vi "RESTful Qualify Routing Templates.vi"(9 "qualified VI names":string[](array[string]), 10 "relative VI paths":path[](array[path]), 11 "Routing Templates":T1[](array[typedef])) -> (3 "Routing Templates out":T1[](array[typedef]))   [LabVIEW 2020]
uses:
  <vilib>/AppBuilder/AB_Classes/RESTful/AB_RESTful_RoutingTemplate.ctl
  <vilib>/AppBuilder/AB_Classes/RESTful/AB_RESTful_RoutingType.ctl
  <vilib>/AppBuilder/AB_Classes/RESTful/AB_RESTful_HTTPMethodType.ctl
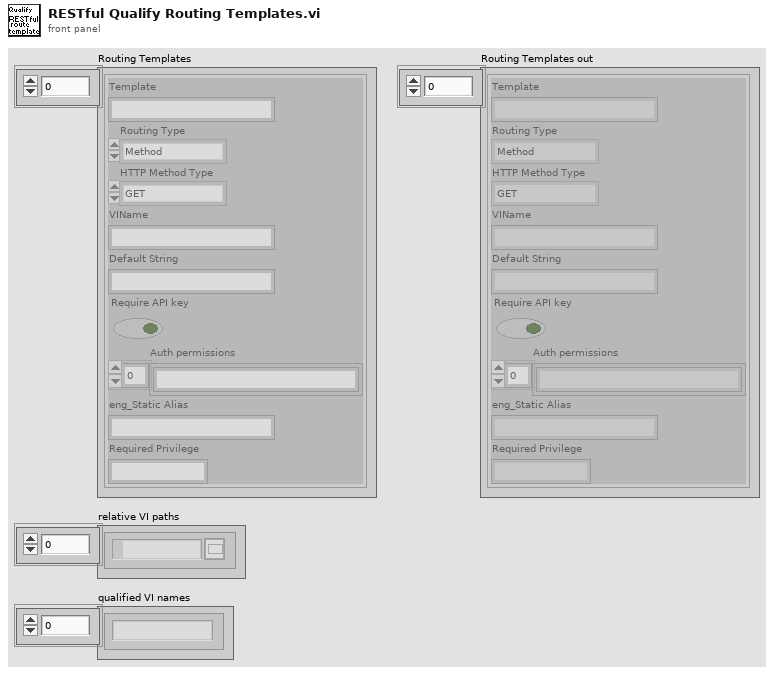
[diagram p1: front panel]
types:
  T1 = typedef "AB_RESTful_RoutingTemplate.ctl" = cluster{"Template":string, "Routing Type":T2, "HTTP Method Type":T3, "VIName":string, "Default String":string, "Require API key":bool, "Auth permissions":string[], "eng_Static Alias":string, "Required Privilege":string}
  T2 = typedef "AB_RESTful_RoutingType.ctl" = enum32{"Method", "Static"}
  T3 = typedef "AB_RESTful_HTTPMethodType.ctl" = enum32{"GET", "POST", "PUT", "DELETE"}
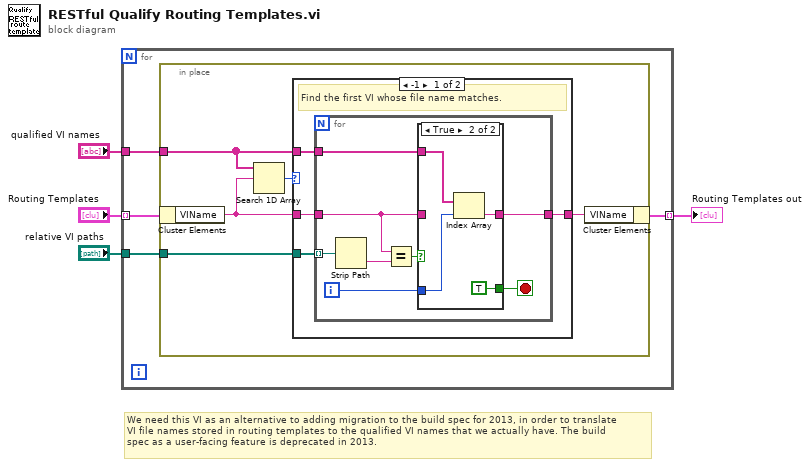
[diagram p0: block diagram]
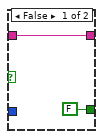
[diagram p2: hidden frame]
diagram:
  # "We need this VI as an alternative to adding migration to the build spec for 2013, in order to translate\nVI file names stored in routing templates to the qualified VI names that we actually have. The build\nspec as a user-facing feature is deprecated in 2013."
  n1 = for {
    tunnel: "Routing Templates" -> [w8] mode=indexing
    tunnel: "qualified VI names" -> [w7]
    tunnel: "relative VI paths" -> [w6]
    tunnel: [w5] -> w4 mode=indexing
    n2 = in-place {
      in-place-border: w7 -> [w9]
      in-place-border: w6 -> [w10]
      n3 = in-place-cluster #1(w8) -> ("VIName"=w12:string)
      n4 = Search 1D Array(1D array=w9, element=w12) -> (index of element=w13:i32)  [unwired: 1 in]
      n5 = case shown="-1" w13 {
        tunnel: w12 -> [w16 w32]
        tunnel: [w14 w32] -> w11
        tunnel: w10 -> [w17 _]
        tunnel: w9 -> [w15 _]
        frame -1 {
          # "Find the first VI whose file name matches."
          n6 = for {
            tunnel: w17 -> [w25] mode=indexing
            tunnel: w16 -> [w19]
            tunnel: w15 -> [w22]
            tunnel: [w20] -> w14
            i -> [w21]
            stop <- w18 stop-if-true
            n7 = Strip Path(path=w25) -> (name=w24:string)  [unwired: 1 out]
            n8 = Equal?(x=w19, y=w24) -> (x = y?=w23:bool)
            n9 = case shown="True" w23 {
              tunnel: w22 -> [_ w31]
              tunnel: w21 -> [_ w30]
              tunnel: [w27 w29] -> w20
              tunnel: w19 -> [w27 _]
              tunnel: [FALSE TRUE] -> w18
              frame False {
              }
              frame True {
                n10 = Index Array(array=w31, index=w30) -> (element=w29:string)
              }
            }
          }
        }
        frame Default {
          # "We matched a qualified VI name."
        }
      }
      n11 = in-place-cluster #1("VIName"=w11) -> (w5:T1)
    }
  }
  "Routing Templates out" <- w4
